vi "Get Rx Start Time.vi"(11 "Framework Performance in":refnum<class "Framework Performance.lvclass">) -> (2 "Rx start time":u32 format="%d us", 3 "Framework Performance out":refnum<class "Framework Performance.lvclass">)   [LabVIEW 2017, in "DSF Core.lvlib" / "Framework Performance.lvclass"]
uses:
  Framework Performance.lvclass
  Framework Performance.lvclass/Framework Performance.ctl
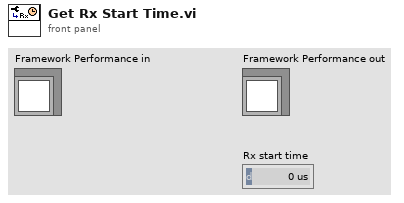
[diagram p1: front panel]
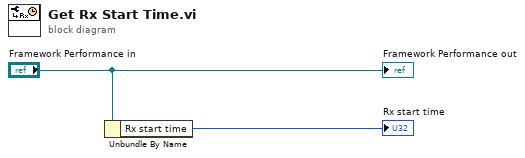
[diagram p0: block diagram]
diagram:
  n1 = Unbundle By Name("Framework Performance in") -> ("Rx start time"=→"Rx start time":u32)
  "Framework Performance out" <- "Framework Performance in"
